vi "SetMixerFrequency.vi"(8 "error in (no error)":errorcluster, 10 "Mixer freq [MHz]":dbl, 11 "ScopeBase In":refnum<class "ScopeBase.lvclass">) -> (0 "error out":errorcluster, 3 "ScopeBase Out":refnum<class "ScopeBase.lvclass">)   [LabVIEW 2018, in "ScopeBase.lvclass"]
uses:
  ScopeBase.lvclass
  ScopeBase.lvclass/ScopeBase.ctl
  <vilib>/Utility/error.llb/Error Cluster From Error Code.vi
  <vilib>/rvi/errors/niLvFpgaAdjustHostInterfaceError.vi
  <vilib>/rvi/interface/nirviReadWriteControl/nirviReadWriteControl.xnode
  FpgaRef/FpgaRefBase/Common FPGA ref.ctl
  FpgaRef/FpgaRefBase/FpgaRefBase.lvclass
  NiFpgaLv.dll
  <vilib>/rvi/interface/Simulation/niFpgaSimulationCallBeginRW.vi
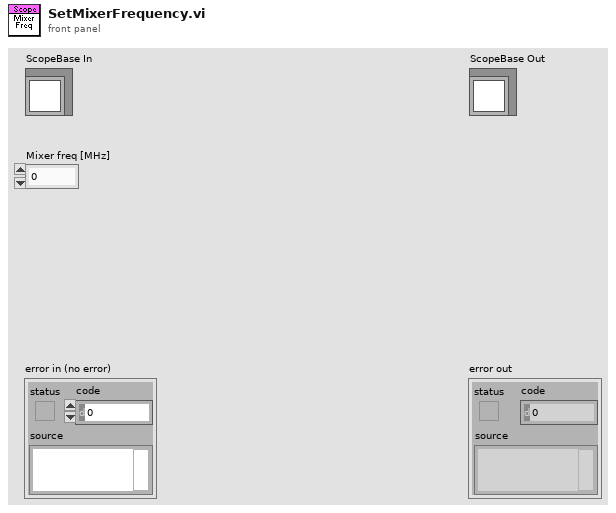
[diagram p1: front panel]
types:
  T1 = typedef "Common FPGA ref.ctl" = refnum<k20>
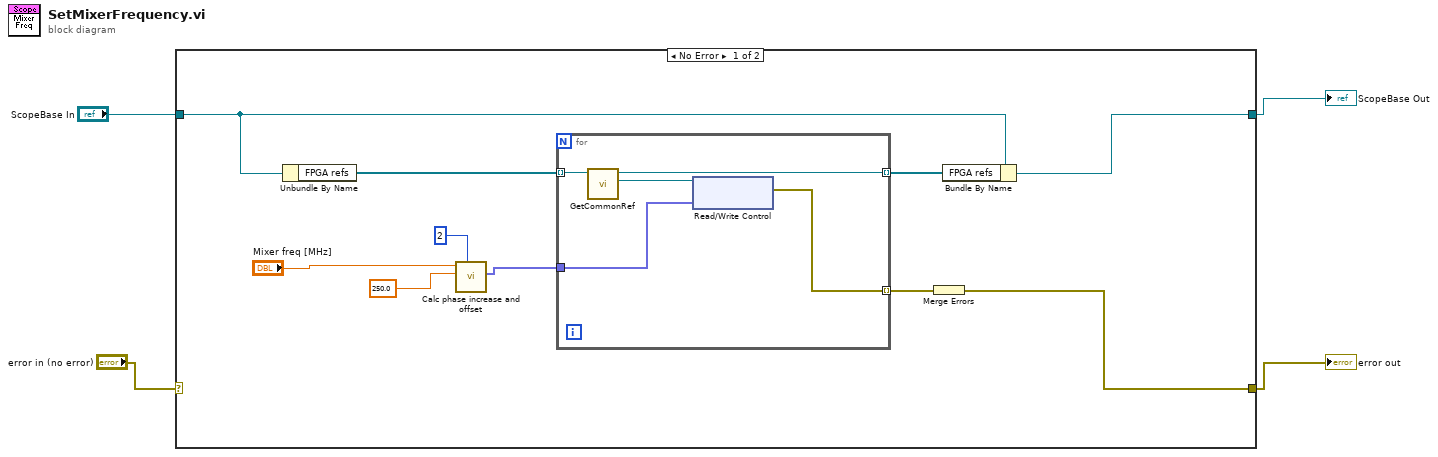
[diagram p0: block diagram]
diagram:
  n1 = case shown="No Error" "error in (no error)" {
    selector: "error in (no error)" -> [_ w21]
    tunnel: [w5 w21] -> w2
    tunnel: [w11 w20] -> w3
    tunnel: "ScopeBase In" -> [w12 w20]
    frame No Error {
      n2 = Unbundle By Name(w12) -> ("FPGA refs"=w14:refnum<class "FpgaRefBase.lvclass">[])
      n3 = call "Calc phase increase and offset.vi"("# of DDS"=2, "fclk (MHz)"=250.0 ("fclk (800MHz)"), "f_generated (MHz)"="Mixer freq [MHz]") -> ("Phase out"=w7:fxp<+,64,64>[])  [unwired: 6 in, 2 out]
      n4 = for {
        tunnel: w7 -> [w19]
        tunnel: w14 -> [w18] mode=indexing
        tunnel: [w16] -> w13 mode=indexing
        tunnel: [w15] -> w6 mode=indexing
        n5 = call-dynamic "GetCommonRef.vi"("FpgaRefBase in"=w18) -> ("Common ref"=w17:T1, "FpgaRefBase out"=w16:refnum<class "FpgaRefBase.lvclass">)  [unwired: 8 in, 1 out]
        n6 = xnode "Read/Write Control"("FPGA VI Reference In"=w17, "Phase input"=w19) -> ("error out"=w15:errorcluster)  [unwired: 1 in, 1 out]
      }
      n7 = Merge Errors(w6) -> (w5:errorcluster)
      n8 = Bundle By Name(cluster=w12, "FPGA refs"=w13) -> (w11:refnum<class "ScopeBase.lvclass">)
    }
    frame Error {
    }
  }
  "error out" <- w2
  "ScopeBase Out" <- w3
